vi "Configure Backlash Factor.vi"(7 "Pump ID (0:A)":T1, 8 "error in (no error)":errorcluster, 10 "Backlash Correction (0 uL)":dbl, 11 "VISA resource in":refnum<visa-resource-name>) -> (0 "error out":errorcluster, 3 "VISA resource out":refnum<visa-resource-name>)   [LabVIEW 2015, in "Global FIA milliGAT.lvlib"]
uses:
  Global FIA milliGAT.lvlib
  Private/Pump Parameter.ctl
  Utility/Pump Address.ctl
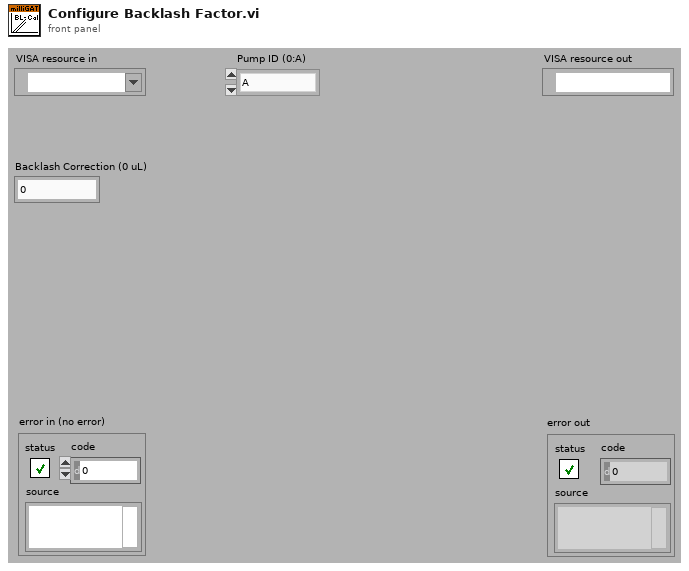
[diagram p1: front panel]
types:
  T1 = typedef "Global FIA milliGAT.lvlib/Pump Address.ctl" = enum16{"A", "B", "C", "D", "E", "F", "G", "H", "I", "J", "K", "L", "M", "N", "O", "P", "Q", "R", "S", "T", "U", "V", "W", "X", "Y", "Z", "a", "b", "c", "d", "e", "f", "g", "h", "i", "j", "k", "l", "m", "n", "o", "p", "q", "r", "s", "t", "u", "v", "w", "x", "y", "z", "0", "1", "2", "3", "4", "5", "6", "7", "8", "9"}
  T2 = typedef "Global FIA milliGAT.lvlib/Pump Parameter.ctl" = enum16{"Enabled", "EU", "EU Calibration Factor", "Fixed Asp or Disp", "Starting Position", "Starting Flow", "Peak Flow", "Flow Acceleration", "Flow Deceleration", "Session Volume", "Max Pressure", "Backlash (usteps)", "BL Calibration Factor", "BL Correction Enabled", "Min Flow", "Max Flow", "Min Acceleration", "Max Acceleration", "Service Volume", "Life Volume"}
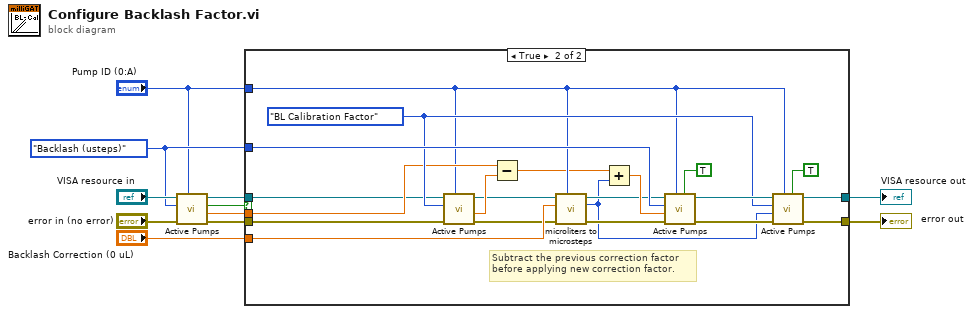
[diagram p0: block diagram]
diagram:
  w5 = Pump_Parameter."Backlash (usteps)" ("Parameter")
  n1 = call "Active Pumps.vi"("Pump ID (0:A)"="Pump ID (0:A)", "error in (no error)"="error in (no error)", "Parameter"=w5, "VISA resource in"="VISA resource in") -> ("error out"=w1:errorcluster, "Value out"=w6:dbl, "Found"=w7:bool, "VISA resource out"=w2:refnum<visa-resource-name>)  [unwired: 4 in]
  n2 = case shown="True" w7 {
    tunnel: [w13 w34] -> w9
    tunnel: [w12 w33] -> w8
    tunnel: "Pump ID (0:A)" -> [_ w22]
    tunnel: "Backlash Correction (0 uL)" -> [_ w23]
    tunnel: w6 -> [_ w24]
    tunnel: w1 -> [w13 w19]
    tunnel: w2 -> [w12 w20]
    tunnel: w5 -> [_ w28]
    frame False {
      # "Not Found"
    }
    frame True {
      w25 = Pump_Parameter."BL Calibration Factor" ("Parameter")
      # "Subtract the previous correction factor\nbefore applying new correction factor."
      n3 = call "Active Pumps.vi"("Pump ID (0:A)"=w22, "error in (no error)"=w19, "Parameter"=w25, "VISA resource in"=w20) -> ("error out"=w18:errorcluster, "Value out"=w26:dbl, "VISA resource out"=w17:refnum<visa-resource-name>)  [unwired: 4 in, 1 out]
      n4 = Subtract(x=w24, y=w26) -> (x-y=w21:dbl)
      n5 = call "microliters to microsteps.vi"("Pump ID (0:A)"=w22, "error in (no error)"=w18, "Microliters (0)"=w23, "VISA resource in"=w17) -> ("error out"=w15:errorcluster, "Microsteps (I32)"=w14:i32, "VISA resource out"=w16:refnum<visa-resource-name>)  [unwired: 4 in, 1 out]
      n6 = Add(x=w21, y=w14) -> (x+y=w29:dbl)
      n7 = call "Active Pumps.vi"("Action (F:Read)"=TRUE, "Pump ID (0:A)"=w22, "error in (no error)"=w15, "Value in"=w29, "Parameter"=w28, "VISA resource in"=w16) -> ("error out"=w31:errorcluster, "VISA resource out"=w30:refnum<visa-resource-name>)  [unwired: 2 in, 2 out]
      n8 = call "Active Pumps.vi"("Action (F:Read)"=TRUE, "Pump ID (0:A)"=w22, "error in (no error)"=w31, "Value in"=w14, "Parameter"=w25, "VISA resource in"=w30) -> ("error out"=w34:errorcluster, "VISA resource out"=w33:refnum<visa-resource-name>)  [unwired: 2 in, 2 out]
    }
  }
  "VISA resource out" <- w8
  "error out" <- w9
